vi "Example - Basic IPS-SA Legacy.vi"(0 "Connection Details":T5={"VISA resource name"="", "Comms Layer"=enum."ISOBus - RS-232", "Serial Configuration"={"Baud Rate"=115200, "Parity"=0, "Data Bits"=8, "Stop Bits"=10, "Flow Control"=0}, "ISOBUS address"=-1} {"Serial Configuration"."Flow Control" items=["None", "XON/XOFF", "RTS/CTS", "XON/XOFF & RTS/CTS", "DTR/DSR", "XON/XOFF & DTR/DSR"]; "Serial Configuration"."Stop Bits" items=["1.0"=10, "2.0"=20]; "Serial Configuration"."Data Bits" items=["7"=7, "8"=8]; "Serial Configuration"."Parity" items=["None", "Odd", "Even"]; "Serial Configuration"."Baud Rate" items=["300"=300, "600"=600, "1200"=1200, "2400"=2400, "4800"=4800, "9600"=9600, "14400"=14400, "19200"=19200, "38400"=38400, "57600"=57600, "115200"=115200]}, 4 "stop":bool, 6 "Ramp Controls":T6 {"Target Rate (T/min)" format="%_5g"; "Target Field (T)" format="%_5g"; "Target Rate (A/min)" format="%_5g"; "Target Current (A)" format="%_5g"}, 7 "Display Units":bool caption="AMP/TESLA", 8 "Magnet Controls":T7, 9 "SWITCH\nHEATER":bool, 11 "Sw Delay (s)":dbl=30.0 caption="Time Target (s)") -> (13 "SW HTR\nCONFIRM":bool, 14 "Output Current (A)":dbl format="%.4g", 15 "Magnet Current (A)":dbl format="%.4g", 16 "Output Voltage (V)":dbl format="%.4f", 19 "error out":errorcluster)   [LabVIEW 2013]
uses:
  <instrlib>/Mercury iXX/Public/Controls/Comms Transport Layer.ctl
  <instrlib>/Mercury iXX/Public/Controls/Serial Settings.ctl
  <instrlib>/Mercury iXX/Public/Controls/ISOBus Address.ctl
  <instrlib>/Mercury iXX/Mercury iXX.lvlib
  <instrlib>/Mercury iXX/Public/Libraries/Temperature/Signals/Read/Temperature (Read).vi
  <instrlib>/Mercury iXX/Public/Libraries/Temperature.lvlib
panel:
  out "Switch TS":timestamp
  out "Sentinel":bool
  in  "Tab Control":T1(tab)
  in  "VISA timeout":u32=1000
  in  "Use VISA?":bool
  in  "Interval between messages (ms)":i16=100
  out "Sys_time_stamp":timestamp
  in  "Secondary address":string="1"
  in  "Primary address":string="22"
  in  "Number of units":dbl=1.0 min=1.0 max=10.0 step=1.0 format="%#.0g"
  in  "Level Card?":bool caption="AMP/TESLA"
  out "N2 Level (%)":dbl format="%.1g"
  out "He Level (%)":dbl format="%.1g"
  out "Mode":string
  out "Voltage (V)":dbl(knob) scale=-10.0..10.0
  out "Current (A)":dbl(knob) scale=-60.0..60.0
  out "Elapsed\nTime (s)":dbl caption="Elapsed Time (s)"
  out "Magnet Centre Field (T)":dbl format="%.4f"
  out "Output (T) (Field equivalent)":dbl format="%.4f"
  out "Status":string
  in  "Log file:":string="C:\\temp\\iPS_data.lvm"
  in  "Log Data?":bool
  in  "Plot Data?":bool
  out "Waveform Chart":T8(graph)
  # "Switch Controls"
  # "MercuryiPS-Legacy-VI"
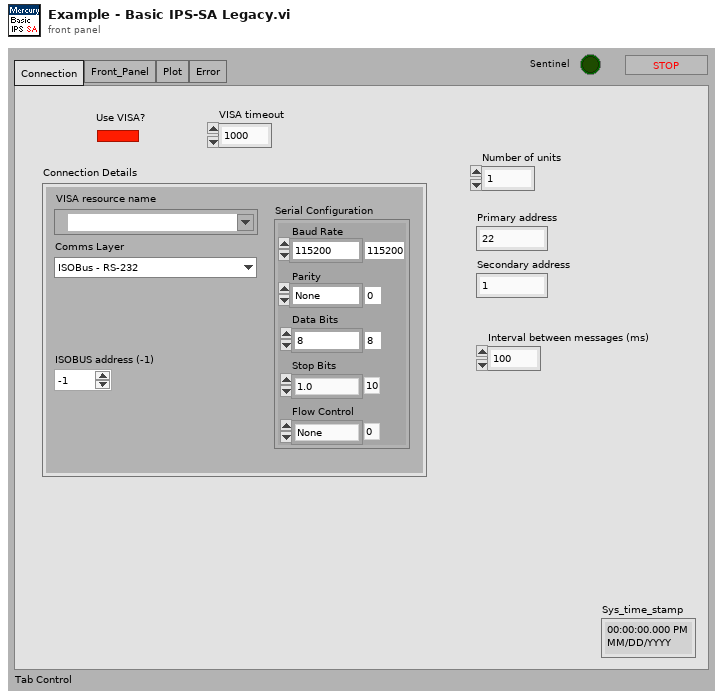
[diagram p1: front panel]
types:
  T1 = enum32{"Connection", "Front_Panel", "Plot", "Error"}
  T2 = typedef "Mercury iXX.lvlib/Comms Transport Layer.ctl" = enum16{"Ethernet TCP/IP", "USB", "ISOBus - RS-232", "GPIB"}
  T3 = typedef "Mercury iXX.lvlib/Serial Settings.ctl" = cluster{"Baud Rate":u32, "Parity":u16, "Data Bits":u16, "Stop Bits":u16, "Flow Control":u16}
  T4 = typedef "Mercury iXX.lvlib/ISOBus Address.ctl" = i32
  T5 = cluster{"VISA resource name":refnum<visa-resource-name>, "Comms Layer":T2, "Serial Configuration":T3, "ISOBUS address":T4}
  T6 = cluster{"Target Current (A)":dbl, "Target Rate (A/min)":dbl, "Target Field (T)":dbl, "Target Rate (T/min)":dbl}
  T7 = cluster{"CLAMP":bool, "HOLD":bool, "TO SET":bool, "TO ZERO":bool}
  T8 = cluster{"Current":dbl, "Persistant Current":dbl, "Voltage":dbl, "Temperature":dbl}
  T9 = cluster{"Current (A) 2":dbl, "Magnet Current (A) 2":dbl, "Voltage (V) 2":dbl, "Temperature":dbl}
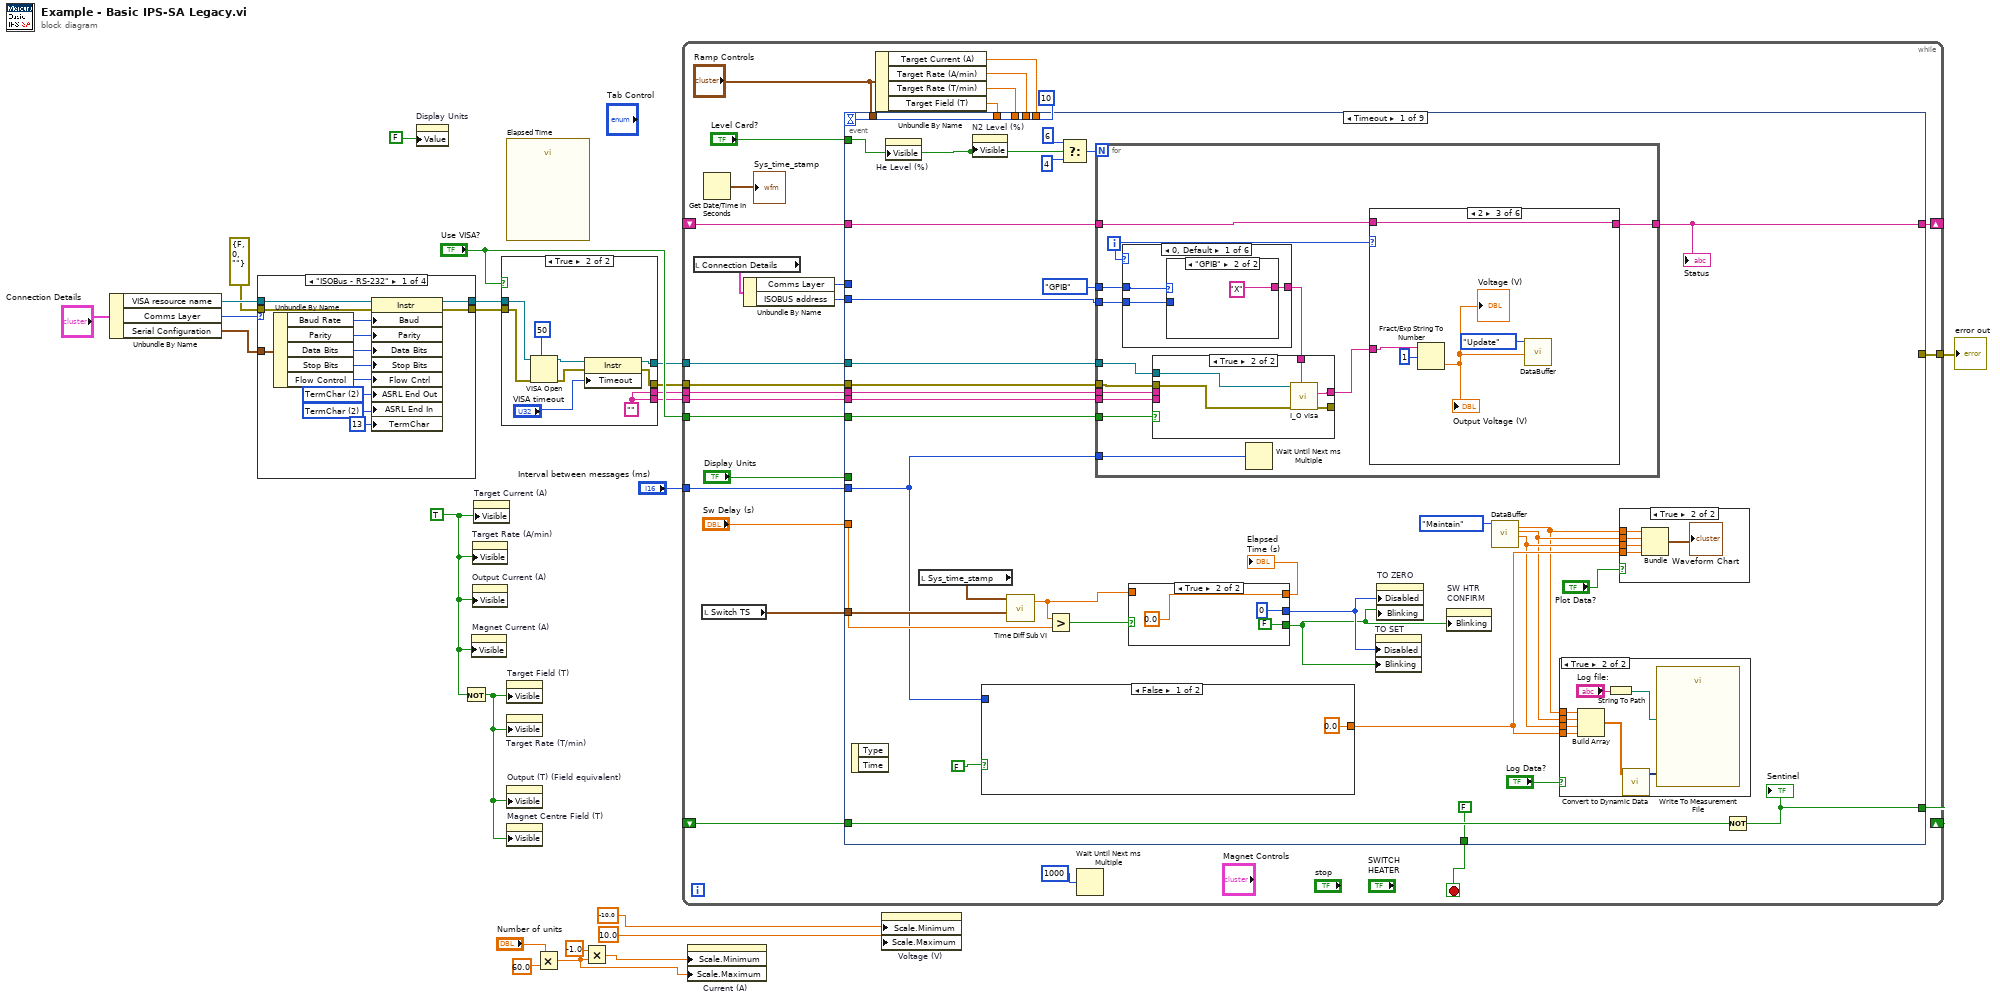
[diagram p0: block diagram]
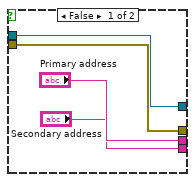
[diagram p2: hidden frame]
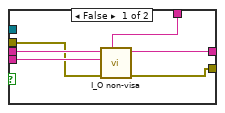
[diagram p6: hidden frame]
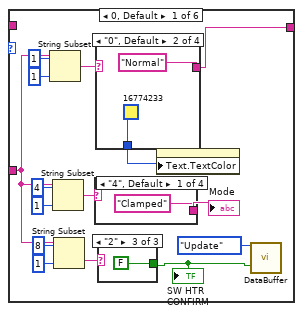
[diagram p7: hidden frame]
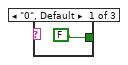
[diagram p8: hidden frame]
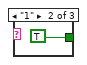
[diagram p9: hidden frame]
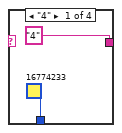
[diagram p10: hidden frame]
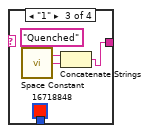
[diagram p11: hidden frame]
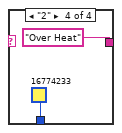
[diagram p12: hidden frame]
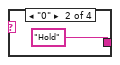
[diagram p13: hidden frame]
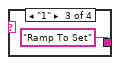
[diagram p14: hidden frame]
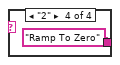
[diagram p15: hidden frame]
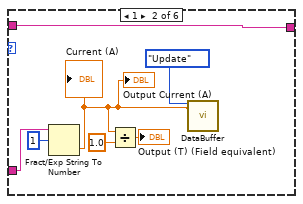
[diagram p16: hidden frame]
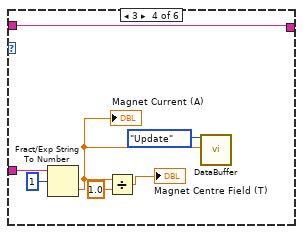
[diagram p17: hidden frame]
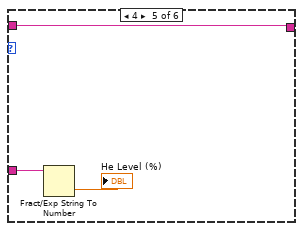
[diagram p18: hidden frame]
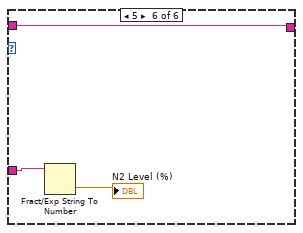
[diagram p19: hidden frame]
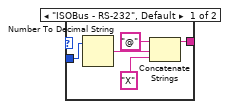
[diagram p20: hidden frame]
diagram:
  w23 = TRUE ("Visible")
  n1 = Unbundle By Name("Connection Details") -> ("VISA resource name"=w13:refnum<visa-resource-name>, "Comms Layer"=w15:T2, "Serial Configuration"=w14:T3)
  n2 = case shown="\"ISOBus - RS-232\"" w15 {
    tunnel: w14 -> [w36 _ _ _]
    tunnel: w13 -> [w37 w39 w41 w43]
    tunnel: errorcluster {"status"=FALSE, "code"=0, "source"=""} ("error in (no error)") -> [w28 w38 w40 w42]
    tunnel: [w27 w39 w41 w43] -> w10
    tunnel: [w26 w38 w40 w42] -> w9
    frame "ISOBus - RS-232" {
      w29 = u16 2 items=["None", "Last Bit", "TermChar"] ("Serial Settings:End Mode for Reads")
      w30 = u16 2 items=["None", "Last Bit", "TermChar", "Break"] ("Serial Settings:End Mode for Writes")
      n3 = Unbundle By Name(w36) -> ("Baud Rate"=w35:u32, "Parity"=w34:u16, "Data Bits"=w33:u16, "Stop Bits"=w32:u16, "Flow Control"=w31:u16)
      n4 = property class="Instr"(reference=w37, error in=w28, "Baud"=w35, "Parity"=w34, "Data Bits"=w33, "Stop Bits"=w32, "Flow Cntrl"=w31, "ASRL End Out"=w30, "ASRL End In"=w29, "TermChar"=u8 13 ("Message Based Settings:Termination Character")) -> (reference out=w27:refnum<visa-resource-name>, error out=w26:errorcluster)
    }
    frame "USB" {
    }
    frame "Ethernet TCP/IP" {
    }
    frame "GPIB" {
    }
  }
  n5 = property on="Display Units" class="Bool (strict)"("Value"=FALSE ("AMP/TESLA")) -> ()  [unwired: 2 in, 2 out]
  n6 = Not(x=w23) -> (.not. x?=w22:bool)
  n7 = property on="Magnet Current (A)" class="DigNum (strict)"("Visible"=w23) -> ()  [unwired: 2 in, 2 out]
  n8 = property on="Target Rate (A/min)" class="DigNum (strict)"("Visible"=w23) -> ()  [unwired: 2 in, 2 out]
  n9 = property on="Output Current (A)" class="DigNum (strict)"("Visible"=w23) -> ()  [unwired: 2 in, 2 out]
  n10 = property on="Target Current (A)" class="DigNum (strict)"("Visible"=w23) -> ()  [unwired: 2 in, 2 out]
  n11 = case shown="True" "Use VISA?" {
    tunnel: w10 -> [w47 w56]
    tunnel: w9 -> [w46 w55]
    tunnel: [w47 w50] -> w5
    tunnel: [w46 w49] -> w6
    tunnel: ["Primary address" w54] -> w8
    tunnel: ["Secondary address" w54] -> w7
    frame False {
    }
    frame True {
      w54 = ""
      n12 = VISA Open(timeout (0)=u32 50 ("VISA Open timeout (0)"), error in (no error)=w55, VISA resource name=w56) -> (VISA resource name=w53:refnum<visa-resource-name>, error out=w52:errorcluster)  [unwired: 2 in]
      n13 = property class="Instr"(reference=w53, error in=w52, "Timeout"="VISA timeout") -> (reference out=w50:refnum<visa-resource-name>, error out=w49:errorcluster)
    }
  }
  n14 = call "Elapsed Time"() -> ()  [unwired: 12 in, 8 out]
  n15 = property on="Target Field (T)" class="DigNum (strict)"("Visible"=w22) -> ()  [unwired: 2 in, 2 out]
  n16 = property on="Target Rate (T/min)" class="DigNum (strict)"("Visible"=w22) -> ()  [unwired: 2 in, 2 out]
  n17 = property on="Output (T) (Field equivalent)" class="DigNum (strict)"("Visible"=w22) -> ()  [unwired: 2 in, 2 out]
  n18 = property on="Magnet Centre Field (T)" class="DigNum (strict)"("Visible"=w22) -> ()  [unwired: 2 in, 2 out]
  n19 = Multiply(x="Number of units", y=60.0) -> (x*y=w18:dbl)
  n20 = Multiply(x=-1.0, y=w18) -> (x*y=w19:dbl)
  n21 = while {
    shift-right: [w80] -> _
    shift-left: _ -> [w81]
    tunnel: [w78] -> w4
    tunnel: "Interval between messages (ms)" -> [w71]
    shift-right: [w66] -> _
    shift-left: _ -> [w70]
    tunnel: "Use VISA?" -> [w65]
    tunnel: w7 -> [w64]
    tunnel: w8 -> [w63]
    tunnel: w6 -> [w62]
    tunnel: w5 -> [w61]
    stop <- w79 stop-if-true
    n22 = local read "Connection Details"() -> (w60:T5)
    n23 = local read "Switch TS"() -> (w69:timestamp)
    n24 = Get Date/Time In Seconds() -> (seconds since 1Jan1904=→"Sys_time_stamp":timestamp)
    n25 = Unbundle By Name(w60) -> ("Comms Layer"=w59:T2, "ISOBUS address"=w58:T4)
    n26 = Unbundle By Name("Ramp Controls") -> ("Target Current (A)"=w74:dbl, "Target Rate (A/min)"=w75:dbl, "Target Rate (T/min)"=w73:dbl, "Target Field (T)"=w72:dbl)
    n27 = event shown="[0] Timeout" {
      selector: _ -> [_ _ _ _ _ _ _ _ _]
      dyn-events: _ -> [_ _ _ _ _ _ _ _ _]
      timeout: 10 -> [_ _ _ _ _ _ _ _ _]
      tunnel: w81 -> [w116 w294 w342 w390 w438 w486 w541 w775 _]
      tunnel: [w115 w294 w342 w390 w438 w486 w541 w775 _] -> w80
      tunnel: [_ _ _ _ _ _ _ _ w780] -> w78
      tunnel: [FALSE FALSE FALSE FALSE FALSE FALSE FALSE TRUE _] -> w79
      tunnel: "Sw Delay (s)" -> [w113 _ _ _ _ _ _ _ _]
      tunnel: "Display Units" -> [_ _ _ _ _ _ w540 _ w779]
      tunnel: w75 -> [_ _ _ _ _ _ w539 _ _]
      tunnel: w74 -> [_ _ _ _ _ _ w538 _ _]
      tunnel: w73 -> [_ _ _ _ _ _ w537 _ _]
      tunnel: w72 -> [_ _ _ _ _ _ w536 _ _]
      tunnel: w71 -> [w96 w291 w333 w381 w429 w484 w535 _ _]
      tunnel: w70 -> [w100 _ _ _ _ _ _ _ _]
      tunnel: w69 -> [w105 _ _ _ _ _ _ _ _]
      tunnel: "Ramp Controls" -> [_ _ _ _ _ _ w534 _ _]
      tunnel: "Level Card?" -> [w93 _ _ _ _ _ _ _ _]
      tunnel: [w101 _ _ _ _ _ _ _ _] -> w66
      tunnel: w65 -> [w99 w285 w334 w382 w430 w474 w530 _ _]
      tunnel: w64 -> [w98 w283 w331 w379 w427 w473 w528 _ _]
      tunnel: w63 -> [w97 w281 w329 w377 w425 w472 w529 _ _]
      tunnel: w62 -> [w95 _ _ _ _ _ _ _ w777]
      tunnel: w61 -> [w94 w279 w327 w375 w423 w471 w527 _ _]
      tunnel: w59 -> [_ w290 w336 w384 w432 w476 w532 _ _]
      tunnel: w58 -> [w85 w287 w335 w383 w431 w475 w531 _ _]
      event Timeout {
        n28 = event-data() -> ()  [unwired: 3 out]
        n29 = property on="He Level (%)" class="DigNum (strict)"("Visible"=w93) -> ()  [unwired: 2 in, 2 out]
        n30 = local read "Sys_time_stamp"() -> (w103:timestamp)
        n31 = property on="N2 Level (%)" class="DigNum (strict)"("Visible"=w93) -> ()  [unwired: 2 in, 2 out]
        n32 = case shown="False" FALSE {
          tunnel: [0.0 ("Temperature") w255] -> w106
          tunnel: w96 -> [_ w253]
          frame False {
          }
          frame True {
            n33 = flat-sequence {
              tunnel: w253 -> [w256]
              tunnel: [w257] -> w254
              tunnel: [w259] -> w255
              tunnel: w254 -> [w259]
              tunnel: w253 -> [w258]
              frame #0 {
                n34 = Wait (ms)(milliseconds to wait=w256) -> ()  [unwired: 1 out]
              }
              frame #1 {
                n35 = call-poly <instrlib>:"Signals (Read).vi"() -> ("Temperature"=w257:dbl)  [unwired: 7 in, 4 out]
              }
              frame #2 {
                n36 = Wait (ms)(milliseconds to wait=w258) -> ()  [unwired: 1 out]
              }
            }
          }
        }
        n37 = call <instrlib>:"Time Diff Sub VI.vi"("Start Time Stamp"=w105, "Current Time Stamp"=w103) -> ("Time Diff"=w104:dbl)  [unwired: 2 in, 1 out]
        n38 = Greater?(x=w104, y=w113) -> (0:w112:bool)
        n39 = Select(t=6, s=w93, f=4) -> (s? t:f=w90:i32)
        n40 = for {
          N: w90 -> [_]
          tunnel: [w126] -> w101
          tunnel: w100 -> [w125]
          tunnel: w99 -> [w124]
          tunnel: w98 -> [w123]
          tunnel: w97 -> [w122]
          tunnel: w96 -> [w121]
          tunnel: w95 -> [w120]
          tunnel: w94 -> [w119]
          tunnel: Comms_Transport_Layer."GPIB" ("Comms Layer") -> [w118]
          tunnel: w85 -> [w117]
          i -> [w128]
          n41 = case shown="0, Default" w128 {
            tunnel: [w199 w207 w218 w225 w234 w244] -> w129
            tunnel: w118 -> [w198 w209 w217 w227 w236 w245]
            tunnel: w117 -> [w200 w208 w216 w226 w235 w243]
            frame 0, Default {
              n42 = case shown="\"GPIB\"" w198 {
                tunnel: [w201 "X" ("data to write")] -> w199
                tunnel: w200 -> [w203 _]
                frame "ISOBus - RS-232", Default {
                  n43 = Number To Decimal String(number=w203) -> (decimal integer string=w204:string)  [unwired: 1 in]
                  n44 = Concatenate Strings("@" ("string"), w204, "X" ("data to write")) -> (w201:string)
                }
                frame "GPIB" {
                }
              }
            }
            frame 1 {
              n45 = case shown="\"ISOBus - RS-232\", Default" w209 {
                tunnel: [w210 "R0" ("data to write")] -> w207
                tunnel: w208 -> [w212 _]
                frame "ISOBus - RS-232", Default {
                  n46 = Number To Decimal String(number=w212) -> (decimal integer string=w213:string)  [unwired: 1 in]
                  n47 = Concatenate Strings("@" ("string"), w213, "R0" ("data to write")) -> (w210:string)
                }
                frame "GPIB" {
                }
              }
            }
            frame 2 {
              n48 = case shown="\"ISOBus - RS-232\", Default" w217 {
                tunnel: [w219 "R1" ("data to write")] -> w218
                tunnel: w216 -> [w221 _]
                frame "ISOBus - RS-232", Default {
                  n49 = Number To Decimal String(number=w221) -> (decimal integer string=w222:string)  [unwired: 1 in]
                  n50 = Concatenate Strings("@" ("string"), w222, "R1" ("data to write")) -> (w219:string)
                }
                frame "GPIB" {
                }
              }
            }
            frame 3 {
              n51 = case shown="\"ISOBus - RS-232\", Default" w227 {
                tunnel: [w228 "R2" ("data to write")] -> w225
                tunnel: w226 -> [w230 _]
                frame "ISOBus - RS-232", Default {
                  n52 = Number To Decimal String(number=w230) -> (decimal integer string=w231:string)  [unwired: 1 in]
                  n53 = Concatenate Strings("@" ("string"), w231, "R2" ("data to write")) -> (w228:string)
                }
                frame "GPIB" {
                }
              }
            }
            frame 4 {
              n54 = case shown="\"GPIB\"" w236 {
                tunnel: [w237 "R10" ("data to write")] -> w234
                tunnel: w235 -> [w239 _]
                frame "ISOBus - RS-232", Default {
                  n55 = Number To Decimal String(number=w239) -> (decimal integer string=w240:string)  [unwired: 1 in]
                  n56 = Concatenate Strings("@" ("string"), w240, "R10" ("data to write")) -> (w237:string)
                }
                frame "GPIB" {
                }
              }
            }
            frame 5 {
              n57 = case shown="\"GPIB\"" w245 {
                tunnel: [w246 "R11" ("data to write")] -> w244
                tunnel: w243 -> [w248 _]
                frame "ISOBus - RS-232", Default {
                  n58 = Number To Decimal String(number=w248) -> (decimal integer string=w249:string)  [unwired: 1 in]
                  n59 = Concatenate Strings("@" ("string"), w249, "R11" ("data to write")) -> (w246:string)
                }
                frame "GPIB" {
                }
              }
            }
          }
          n60 = case shown="True" w124 {
            tunnel: w129 -> [w135 w140]
            tunnel: [w134 w139] -> w127
            tunnel: w123 -> [w133 _]
            tunnel: w122 -> [w132 _]
            tunnel: w120 -> [w130 w138]
            tunnel: w119 -> [_ w137]
            tunnel: [w131 w136] -> _
            frame False {
              n61 = call <instrlib>:"I_O non-visa.vi"("data to write"=w135, "error in"=w130, "Secondary address"=w133, "Primary address"=w132) -> ("error out"=w131:errorcluster, "read data"=w134:string)  [unwired: 6 in]
            }
            frame True {
              n62 = call <instrlib>:"I_O visa.vi"("data to write"=w140, "error in"=w138, "VISA resource name"=w137) -> ("error out"=w136:errorcluster, "read data"=w139:string)  [unwired: 6 in, 1 out]
            }
          }
          n63 = Wait Until Next ms Multiple(millisecond multiple=w121) -> ()  [unwired: 1 out]
          n64 = case shown="2" w128 {
            tunnel: w127 -> [w146 w179 w184 w190 w194 w197]
            tunnel: [w143 w176 w183 w188 w192 w195] -> w126
            tunnel: w125 -> [_ w176 w183 w188 w192 w195]
            frame 0, Default {
              n65 = String Subset(string=w146, offset (0)=1, length (rest)=1 ("length (rest)")) -> (substring=w149:string)
              n66 = String Subset(string=w146, offset (0)=4, length (rest)=1 ("length (rest)")) -> (substring=w151:string)
              n67 = String Subset(string=w146, offset (0)=8, length (rest)=1 ("length (rest)")) -> (substring=w145:string)
              n68 = case shown="\"4\", Default" w151 {
                tunnel: ["Clamped" "Hold" "Ramp To Set" "Ramp To Zero"] -> w150
                frame "4", Default {
                }
                frame "0" {
                }
                frame "1" {
                }
                frame "2" {
                }
              }
              "Mode" <- w150
              n69 = case shown="\"0\", Default" w149 {
                tunnel: ["4" "Normal" w164 "Over Heat"] -> w143
                tunnel: [u32 16774233 ("Text.Text Colors:Text Color") u32 16774233 ("Text.Text Colors:Text Color") u32 16718848 ("Text.Text Colors:Text Color") u32 16774233 ("Text.Text Colors:Text Color")] -> w144
                frame "4" {
                }
                frame "0", Default {
                }
                frame "1" {
                  n70 = call <vilib>:"Space Constant.vi"() -> ("String"=w165:string)
                  n71 = Concatenate Strings("Quenched", w165) -> (w164:string)
                }
                frame "2" {
                }
              }
              n72 = case shown="\"2\"" w145 {
                tunnel: [FALSE TRUE FALSE] -> w142
                frame "0", Default {
                }
                frame "1" {
                }
                frame "2" {
                }
              }
              "SW HTR\nCONFIRM" <- w142
              n73 = property on="Status" class="Str"("Text.TextColor"=w144) -> ()  [unwired: 2 in, 2 out]
              n74 = call <instrlib>:"DataBuffer.vi"("Enum"=enum16{"Maintain", "Update", "Initialise"}."Update", "Switch Htr State"=w142) -> ()  [unwired: 14 in, 4 out]
            }
            frame 1 {
              n75 = Fract/Exp String To Number(string=w179, offset=1) -> (number=w173:dbl)  [unwired: 2 in, 1 out]
              "Output Current (A)" <- w173
              "Current (A)" <- w173
              n76 = Divide(x=w173, y=1.0) -> (x/y=→"Output (T) (Field equivalent)":dbl)
              n77 = call <instrlib>:"DataBuffer.vi"("Enum"=enum16{"Maintain", "Update", "Initialise"}."Update", "Current (A)"=w173) -> ()  [unwired: 14 in, 4 out]
            }
            frame 2 {
              n78 = Fract/Exp String To Number(string=w184, offset=1) -> (number=w182:dbl)  [unwired: 2 in, 1 out]
              "Voltage (V)" <- w182
              "Output Voltage (V)" <- w182
              n79 = call <instrlib>:"DataBuffer.vi"("Enum"=enum16{"Maintain", "Update", "Initialise"}."Update", "Voltage (V)"=w182) -> ()  [unwired: 14 in, 4 out]
            }
            frame 3 {
              n80 = Fract/Exp String To Number(string=w190, offset=1) -> (number=w187:dbl)  [unwired: 2 in, 1 out]
              "Magnet Current (A)" <- w187
              n81 = Divide(x=w187, y=1.0) -> (x/y=→"Magnet Centre Field (T)":dbl)
              n82 = call <instrlib>:"DataBuffer.vi"("Enum"=enum16{"Maintain", "Update", "Initialise"}."Update", "Magnet Current (A)"=w187) -> ()  [unwired: 14 in, 4 out]
            }
            frame 4 {
              n83 = Fract/Exp String To Number(string=w194) -> (number=→"He Level (%)":dbl)  [unwired: 3 in, 1 out]
            }
            frame 5 {
              n84 = Fract/Exp String To Number(string=w197) -> (number=→"N2 Level (%)":dbl)  [unwired: 3 in, 1 out]
            }
          }
        }
        "Status" <- w101
        n85 = case shown="True" w112 {
          tunnel: [w275 0.0 ("Elapsed\nTime (s)")] -> w111
          tunnel: w104 -> [w275 _]
          tunnel: [TRUE ("Blinking") FALSE ("Blinking")] -> w109
          tunnel: [u8 1 ("Disabled") u8 0 ("Disabled")] -> w110
          frame False {
          }
          frame True {
          }
        }
        "Elapsed\nTime (s)" <- w111
        n86 = property on="TO SET" class="Bool"("Disabled"=w110, "Blinking"=w109) -> ()  [unwired: 2 in, 2 out]
        n87 = property on="TO ZERO" class="Bool"("Disabled"=w110, "Blinking"=w109) -> ()  [unwired: 2 in, 2 out]
        n88 = property on="SW HTR\nCONFIRM" class="Bool (strict)"("Blinking"=w109) -> ()  [unwired: 2 in, 2 out]
        n89 = call <instrlib>:"DataBuffer.vi"("Enum"=enum16{"Maintain", "Update", "Initialise"}."Maintain") -> ("Current (A) 2"=w86:dbl, "Magnet Current (A) 2"=w87:dbl, "Voltage (V) 2"=w88:dbl)  [unwired: 15 in, 1 out]
        n90 = case shown="True" "Log Data?" {
          tunnel: w106 -> [_ w263]
          tunnel: w88 -> [_ w262]
          tunnel: w87 -> [_ w261]
          tunnel: w86 -> [_ w260]
          frame False {
          }
          frame True {
            n91 = Build Array(w260, w261, w262, w263) -> (w265:dbl[])
            n92 = String To Path(string="Log file:") -> (path=w266:path)
            n93 = call "Convert to Dynamic Data"("Array"=w265) -> ("Dynamic Data Type"=w264:dynamicdata)  [unwired: 3 in]
            n94 = call "Write To Measurement File"("Signals"=w264, "Filename"=w266) -> ()  [unwired: 15 in, 3 out]
          }
        }
        n95 = case shown="True" "Plot Data?" {
          tunnel: w106 -> [_ w272]
          tunnel: w88 -> [_ w271]
          tunnel: w87 -> [_ w270]
          tunnel: w86 -> [_ w269]
          frame False {
          }
          frame True {
            n96 = Bundle("Current (A) 2"=w269, "Magnet Current (A) 2"=w270, "Voltage (V) 2"=w271, "Temperature"=w272) -> (→"Waveform Chart":T9)  [unwired: 1 in]
          }
        }
        n97 = Not(x=w116) -> (.not. x?=w115:bool)
        "Sentinel" <- w115
      }
      event "Magnet Controls.HOLD": Mouse Down {
        n98 = event-data() -> ()  [unwired: 7 out]
        n99 = flat-sequence {
          tunnel: [w302] -> w292
          tunnel: w291 -> [w302]
          tunnel: w290 -> [w301]
          tunnel: [w301] -> w289
          tunnel: [w300] -> w288
          tunnel: w287 -> [w300]
          tunnel: [w299] -> w286
          tunnel: w285 -> [w299]
          tunnel: [w298] -> w284
          tunnel: w283 -> [w298]
          tunnel: [w297] -> w282
          tunnel: w281 -> [w297]
          tunnel: [w296] -> w280
          tunnel: w279 -> [w296]
          tunnel: [w310] -> w293
          tunnel: w292 -> [w310]
          tunnel: w289 -> [w308]
          tunnel: w288 -> [w307]
          tunnel: w286 -> [w306]
          tunnel: w284 -> [w305]
          tunnel: w282 -> [w304]
          tunnel: w280 -> [w303]
          tunnel: w293 -> [w326]
          frame #0 {
            n100 = Wait (ms)(milliseconds to wait=w302) -> ()  [unwired: 1 out]
          }
          frame #1 {
            n101 = case shown="\"ISOBus - RS-232\", Default" w308 {
              tunnel: [w312 "A0" ("data to write")] -> w309
              tunnel: w307 -> [w311 _]
              frame "ISOBus - RS-232", Default {
                n102 = Number To Decimal String(number=w311) -> (decimal integer string=w314:string)  [unwired: 1 in]
                n103 = Concatenate Strings("@" ("string"), w314, "A0" ("data to write")) -> (w312:string)
              }
              frame "GPIB" {
              }
            }
            n104 = case shown="True" w306 {
              tunnel: w309 -> [w321 w325]
              tunnel: [w320 w324] -> _
              tunnel: [w319 w323] -> _
              tunnel: w305 -> [w318 _]
              tunnel: w304 -> [w317 _]
              tunnel: w303 -> [_ w322]
              frame False {
                n105 = call <instrlib>:"I_O non-visa.vi"("data to write"=w321, "Secondary address"=w318, "Primary address"=w317) -> ("error out"=w319:errorcluster, "read data"=w320:string)  [unwired: 7 in]
              }
              frame True {
                n106 = call <instrlib>:"I_O visa.vi"("data to write"=w325, "VISA resource name"=w322) -> ("error out"=w323:errorcluster, "read data"=w324:string)  [unwired: 7 in, 1 out]
              }
            }
          }
          frame #2 {
            n107 = Wait (ms)(milliseconds to wait=w326) -> ()  [unwired: 1 out]
          }
        }
      }
      event "Magnet Controls.CLAMP": Mouse Down {
        n108 = event-data() -> ()  [unwired: 7 out]
        n109 = flat-sequence {
          tunnel: [w350] -> w341
          tunnel: w333 -> [w350]
          tunnel: w336 -> [w349]
          tunnel: [w349] -> w340
          tunnel: [w348] -> w339
          tunnel: w335 -> [w348]
          tunnel: [w347] -> w338
          tunnel: w334 -> [w347]
          tunnel: [w346] -> w332
          tunnel: w331 -> [w346]
          tunnel: [w345] -> w330
          tunnel: w329 -> [w345]
          tunnel: [w344] -> w328
          tunnel: w327 -> [w344]
          tunnel: [w358] -> w337
          tunnel: w341 -> [w358]
          tunnel: w340 -> [w356]
          tunnel: w339 -> [w355]
          tunnel: w338 -> [w354]
          tunnel: w332 -> [w353]
          tunnel: w330 -> [w352]
          tunnel: w328 -> [w351]
          tunnel: w337 -> [w374]
          frame #0 {
            n110 = Wait (ms)(milliseconds to wait=w350) -> ()  [unwired: 1 out]
          }
          frame #1 {
            n111 = case shown="\"GPIB\"" w356 {
              tunnel: [w360 "A4" ("data to write")] -> w357
              tunnel: w355 -> [w359 _]
              frame "ISOBus - RS-232", Default {
                n112 = Number To Decimal String(number=w359) -> (decimal integer string=w362:string)  [unwired: 1 in]
                n113 = Concatenate Strings("@" ("string"), w362, "A4" ("data to write")) -> (w360:string)
              }
              frame "GPIB" {
              }
            }
            n114 = case shown="True" w354 {
              tunnel: w357 -> [w369 w373]
              tunnel: [w368 w372] -> _
              tunnel: [w367 w371] -> _
              tunnel: w353 -> [w366 _]
              tunnel: w352 -> [w365 _]
              tunnel: w351 -> [_ w370]
              frame False {
                n115 = call <instrlib>:"I_O non-visa.vi"("data to write"=w369, "Secondary address"=w366, "Primary address"=w365) -> ("error out"=w367:errorcluster, "read data"=w368:string)  [unwired: 7 in]
              }
              frame True {
                n116 = call <instrlib>:"I_O visa.vi"("data to write"=w373, "VISA resource name"=w370) -> ("error out"=w371:errorcluster, "read data"=w372:string)  [unwired: 7 in, 1 out]
              }
            }
          }
          frame #2 {
            n117 = Wait (ms)(milliseconds to wait=w374) -> ()  [unwired: 1 out]
          }
        }
      }
      event "Magnet Controls.TO SET": Mouse Down {
        n118 = event-data() -> ()  [unwired: 7 out]
        n119 = flat-sequence {
          tunnel: [w398] -> w389
          tunnel: w381 -> [w398]
          tunnel: w384 -> [w397]
          tunnel: [w397] -> w388
          tunnel: [w396] -> w387
          tunnel: w383 -> [w396]
          tunnel: [w395] -> w386
          tunnel: w382 -> [w395]
          tunnel: [w394] -> w380
          tunnel: w379 -> [w394]
          tunnel: [w393] -> w378
          tunnel: w377 -> [w393]
          tunnel: [w392] -> w376
          tunnel: w375 -> [w392]
          tunnel: [w406] -> w385
          tunnel: w389 -> [w406]
          tunnel: w388 -> [w404]
          tunnel: w387 -> [w403]
          tunnel: w386 -> [w402]
          tunnel: w380 -> [w401]
          tunnel: w378 -> [w400]
          tunnel: w376 -> [w399]
          tunnel: w385 -> [w422]
          frame #0 {
            n120 = Wait (ms)(milliseconds to wait=w398) -> ()  [unwired: 1 out]
          }
          frame #1 {
            n121 = case shown="\"ISOBus - RS-232\", Default" w404 {
              tunnel: [w408 "A1" ("data to write")] -> w405
              tunnel: w403 -> [w407 _]
              frame "ISOBus - RS-232", Default {
                n122 = Number To Decimal String(number=w407) -> (decimal integer string=w410:string)  [unwired: 1 in]
                n123 = Concatenate Strings("@" ("string"), w410, "A1" ("data to write")) -> (w408:string)
              }
              frame "GPIB" {
              }
            }
            n124 = case shown="True" w402 {
              tunnel: w405 -> [w417 w421]
              tunnel: [w416 w420] -> _
              tunnel: [w415 w419] -> _
              tunnel: w401 -> [w414 _]
              tunnel: w400 -> [w413 _]
              tunnel: w399 -> [_ w418]
              frame False {
                n125 = call <instrlib>:"I_O non-visa.vi"("data to write"=w417, "Secondary address"=w414, "Primary address"=w413) -> ("error out"=w415:errorcluster, "read data"=w416:string)  [unwired: 7 in]
              }
              frame True {
                n126 = call <instrlib>:"I_O visa.vi"("data to write"=w421, "VISA resource name"=w418) -> ("error out"=w419:errorcluster, "read data"=w420:string)  [unwired: 7 in, 1 out]
              }
            }
          }
          frame #2 {
            n127 = Wait (ms)(milliseconds to wait=w422) -> ()  [unwired: 1 out]
          }
        }
      }
      event "Magnet Controls.TO ZERO": Mouse Down {
        n128 = event-data() -> ()  [unwired: 7 out]
        n129 = flat-sequence {
          tunnel: [w446] -> w437
          tunnel: w429 -> [w446]
          tunnel: w432 -> [w445]
          tunnel: [w445] -> w436
          tunnel: [w444] -> w435
          tunnel: w431 -> [w444]
          tunnel: [w443] -> w434
          tunnel: w430 -> [w443]
          tunnel: [w442] -> w428
          tunnel: w427 -> [w442]
          tunnel: [w441] -> w426
          tunnel: w425 -> [w441]
          tunnel: [w440] -> w424
          tunnel: w423 -> [w440]
          tunnel: [w454] -> w433
          tunnel: w437 -> [w454]
          tunnel: w436 -> [w452]
          tunnel: w435 -> [w451]
          tunnel: w434 -> [w450]
          tunnel: w428 -> [w449]
          tunnel: w426 -> [w448]
          tunnel: w424 -> [w447]
          tunnel: w433 -> [w470]
          frame #0 {
            n130 = Wait (ms)(milliseconds to wait=w446) -> ()  [unwired: 1 out]
          }
          frame #1 {
            n131 = case shown="\"ISOBus - RS-232\", Default" w452 {
              tunnel: [w456 "A2" ("data to write")] -> w453
              tunnel: w451 -> [w455 _]
              frame "ISOBus - RS-232", Default {
                n132 = Number To Decimal String(number=w455) -> (decimal integer string=w458:string)  [unwired: 1 in]
                n133 = Concatenate Strings("@" ("string"), w458, "A2" ("data to write")) -> (w456:string)
              }
              frame "GPIB" {
              }
            }
            n134 = case shown="True" w450 {
              tunnel: w453 -> [w465 w469]
              tunnel: [w464 w468] -> _
              tunnel: [w463 w467] -> _
              tunnel: w449 -> [w462 _]
              tunnel: w448 -> [w461 _]
              tunnel: w447 -> [_ w466]
              frame False {
                n135 = call <instrlib>:"I_O non-visa.vi"("data to write"=w465, "Secondary address"=w462, "Primary address"=w461) -> ("error out"=w463:errorcluster, "read data"=w464:string)  [unwired: 7 in]
              }
              frame True {
                n136 = call <instrlib>:"I_O visa.vi"("data to write"=w469, "VISA resource name"=w466) -> ("error out"=w467:errorcluster, "read data"=w468:string)  [unwired: 7 in, 1 out]
              }
            }
          }
          frame #2 {
            n137 = Wait (ms)(milliseconds to wait=w470) -> ()  [unwired: 1 out]
          }
        }
      }
      event "SWITCH\nHEATER": Mouse Down {
        n138 = event-data() -> ()  [unwired: 2 out]
        n139 = call <instrlib>:"DataBuffer.vi"("Enum"=enum16{"Maintain", "Update", "Initialise"}."Maintain") -> ("Current (A) 2"=w479:dbl, "Magnet Current (A) 2"=w478:dbl)  [unwired: 15 in, 2 out]
        n140 = Subtract(x=w479, y=w478) -> (x-y=w481:dbl)
        n141 = Absolute Value(x=w481) -> (abs(x)=w482:dbl)
        n142 = Less?(x=w482, y=0.1) -> (x < y?=w480:bool)
        n143 = case shown="False" w480 {
          selector: w480 -> [_ w490]
          tunnel: [w489 w490] -> w485
          frame False {
            n144 = Two Button Dialog(message="The magnet current is more\nthan 0.1A different to the\nPSU output current.  It is not\nadvisable to switch on the\nswitch heater unless these\ncurrents are equal!") -> (T button?=w489:bool)  [unwired: 2 out]
          }
          frame True {
          }
        }
        n145 = case shown="True" w485 {
          tunnel: w484 -> [_ w497]
          tunnel: w476 -> [_ w496]
          tunnel: w475 -> [_ w495]
          tunnel: w474 -> [_ w494]
          tunnel: w473 -> [_ w493]
          tunnel: w472 -> [_ w492]
          tunnel: w471 -> [_ w491]
          frame False {
          }
          frame True {
            n146 = flat-sequence {
              tunnel: w496 -> [w503]
              tunnel: w495 -> [w502]
              tunnel: w494 -> [w501]
              tunnel: w493 -> [w500]
              tunnel: w492 -> [w499]
              tunnel: w491 -> [w498]
              tunnel: w497 -> [w525]
              frame #0 {
                n147 = call <instrlib>:"DataBuffer.vi"("Enum"=enum16{"Maintain", "Update", "Initialise"}."Maintain") -> ("Sw Htr State 2"=w508:bool)  [unwired: 15 in, 3 out]
                n148 = Select(t="H0" ("data to write"), s=w508, f="H2" ("data to write")) -> (s? t:f=w505:string)
                n149 = case shown="\"ISOBus - RS-232\", Default" w503 {
                  tunnel: [w512 w515] -> w504
                  tunnel: w505 -> [w511 w515]
                  tunnel: w502 -> [w510 _]
                  frame "ISOBus - RS-232", Default {
                    n150 = Number To Decimal String(number=w510) -> (decimal integer string=w514:string)  [unwired: 1 in]
                    n151 = Concatenate Strings("@" ("string"), w514, w511) -> (w512:string)
                  }
                  frame "GPIB" {
                  }
                }
                n152 = case shown="True" w501 {
                  tunnel: [w520 w524] -> _
                  tunnel: [w519 w523] -> _
                  tunnel: w504 -> [w518 w522]
                  tunnel: w500 -> [w516 _]
                  tunnel: w499 -> [w517 _]
                  tunnel: w498 -> [_ w521]
                  frame False {
                    n153 = call <instrlib>:"I_O non-visa.vi"("data to write"=w518, "Secondary address"=w516, "Primary address"=w517) -> ("error out"=w519:errorcluster, "read data"=w520:string)  [unwired: 7 in]
                  }
                  frame True {
                    n154 = call <instrlib>:"I_O visa.vi"("data to write"=w522, "VISA resource name"=w521) -> ("error out"=w523:errorcluster, "read data"=w524:string)  [unwired: 7 in, 1 out]
                  }
                }
              }
              frame #1 {
                n155 = Wait (ms)(milliseconds to wait=w525) -> ()  [unwired: 1 out]
              }
              frame #2 {
                n156 = local read "Sys_time_stamp"() -> (→"Switch TS":timestamp)
              }
            }
          }
        }
      }
      event "Ramp Controls": Value Change {
        n157 = event-data() -> ()  [unwired: 6 out]
        n158 = case shown="False" w540 {
          tunnel: w539 -> [w572 _]
          tunnel: w538 -> [w573 _]
          tunnel: w537 -> [_ w673]
          tunnel: w536 -> [_ w674]
          tunnel: w535 -> [w575 w675]
          tunnel: w534 -> [w570 w694]
          tunnel: [w569 w693] -> w533
          tunnel: w532 -> [w567 w677]
          tunnel: w531 -> [w565 w678]
          tunnel: w530 -> [w563 w676]
          tunnel: w529 -> [w553 w671]
          tunnel: w528 -> [w551 w669]
          tunnel: w527 -> [w555 w667]
          frame False {
            n159 = Divide(x=w573, y=1.0) -> (x/y=w574:dbl)
            n160 = Divide(x=w572, y=1.0) -> (x/y=w571:dbl)
            n161 = flat-sequence {
              tunnel: w573 -> [w588]
              tunnel: [w588] -> w580
              tunnel: [w587] -> w576
              tunnel: w575 -> [w587]
              tunnel: [w586] -> w568
              tunnel: w567 -> [w586]
              tunnel: [w585] -> w566
              tunnel: w565 -> [w585]
              tunnel: [w584] -> w564
              tunnel: w563 -> [w584]
              tunnel: [w583] -> w556
              tunnel: w555 -> [w583]
              tunnel: [w582] -> w554
              tunnel: w553 -> [w582]
              tunnel: [w581] -> w552
              tunnel: w551 -> [w581]
              tunnel: w580 -> [w595]
              tunnel: [w597] -> w577
              tunnel: w576 -> [w597]
              tunnel: w568 -> [w593]
              tunnel: w566 -> [w592]
              tunnel: w564 -> [w594]
              tunnel: [w594] -> w561
              tunnel: [w593] -> w559
              tunnel: [w592] -> w557
              tunnel: w556 -> [w589]
              tunnel: w554 -> [w590]
              tunnel: w552 -> [w591]
              tunnel: [w591] -> w549
              tunnel: [w590] -> w547
              tunnel: [w589] -> w545
              tunnel: [w626] -> w578
              tunnel: w577 -> [w626]
              tunnel: [w625] -> w562
              tunnel: w561 -> [w625]
              tunnel: [w624] -> w560
              tunnel: w559 -> [w624]
              tunnel: [w623] -> w558
              tunnel: w557 -> [w623]
              tunnel: [w622] -> w550
              tunnel: w549 -> [w622]
              tunnel: [w621] -> w548
              tunnel: w547 -> [w621]
              tunnel: [w620] -> w546
              tunnel: w545 -> [w620]
              tunnel: w572 -> [w634]
              tunnel: [w635] -> w579
              tunnel: w578 -> [w635]
              tunnel: w562 -> [w633]
              tunnel: w560 -> [w632]
              tunnel: w558 -> [w631]
              tunnel: w550 -> [w629]
              tunnel: w548 -> [w628]
              tunnel: w546 -> [w627]
              tunnel: w579 -> [w658]
              frame #0 {
                n162 = Wait (ms)(milliseconds to wait=w587) -> ()  [unwired: 1 out]
              }
              frame #1 {
                n163 = case shown="\"ISOBus - RS-232\", Default" w593 {
                  tunnel: [w603 w606] -> w596
                  tunnel: w592 -> [w602 _]
                  tunnel: w595 -> [w600 w609]
                  frame "ISOBus - RS-232", Default {
                    n164 = Number To Decimal String(number=w602) -> (decimal integer string=w605:string)  [unwired: 1 in]
                    n165 = Number To Fractional String(number=w600, precision (6)=i16 4) -> (F-format string=w598:string)  [unwired: 2 in]
                    n166 = Concatenate Strings("@" ("string"), w605, "I" ("data to write"), w598) -> (w603:string)
                  }
                  frame "GPIB" {
                    n167 = Number To Fractional String(number=w609, precision (6)=i16 4) -> (F-format string=w607:string)  [unwired: 2 in]
                    n168 = Concatenate Strings("I" ("data to write"), w607) -> (w606:string)
                  }
                }
                n169 = case shown="True" w594 {
                  tunnel: w596 -> [w615 w619]
                  tunnel: [w614 w618] -> _
                  tunnel: [w613 w617] -> _
                  tunnel: w591 -> [w612 _]
                  tunnel: w590 -> [w611 _]
                  tunnel: w589 -> [_ w616]
                  frame False {
                    n170 = call <instrlib>:"I_O non-visa.vi"("data to write"=w615, "Secondary address"=w612, "Primary address"=w611) -> ("error out"=w613:errorcluster, "read data"=w614:string)  [unwired: 7 in]
                  }
                  frame True {
                    n171 = call <instrlib>:"I_O visa.vi"("data to write"=w619, "VISA resource name"=w616) -> ("error out"=w617:errorcluster, "read data"=w618:string)  [unwired: 7 in, 1 out]
                  }
                }
              }
              frame #2 {
                n172 = Wait (ms)(milliseconds to wait=w626) -> ()  [unwired: 1 out]
              }
              frame #3 {
                n173 = case shown="\"GPIB\"" w632 {
                  tunnel: [w641 w644] -> w630
                  tunnel: w631 -> [w640 _]
                  tunnel: w634 -> [w638 w647]
                  frame "ISOBus - RS-232", Default {
                    n174 = Number To Decimal String(number=w640) -> (decimal integer string=w643:string)  [unwired: 1 in]
                    n175 = Number To Fractional String(number=w638, precision (6)=i16 4) -> (F-format string=w636:string)  [unwired: 2 in]
                    n176 = Concatenate Strings("@" ("string"), w643, "S" ("data to write"), w636) -> (w641:string)
                  }
                  frame "GPIB" {
                    n177 = Number To Fractional String(number=w647, precision (6)=i16 4) -> (F-format string=w645:string)  [unwired: 2 in]
                    n178 = Concatenate Strings("S" ("data to write"), w645) -> (w644:string)
                  }
                }
                n179 = case shown="True" w633 {
                  tunnel: w630 -> [w653 w657]
                  tunnel: [w652 w656] -> _
                  tunnel: [w651 w655] -> _
                  tunnel: w629 -> [w650 _]
                  tunnel: w628 -> [w649 _]
                  tunnel: w627 -> [_ w654]
                  frame False {
                    n180 = call <instrlib>:"I_O non-visa.vi"("data to write"=w653, "Secondary address"=w650, "Primary address"=w649) -> ("error out"=w651:errorcluster, "read data"=w652:string)  [unwired: 7 in]
                  }
                  frame True {
                    n181 = call <instrlib>:"I_O visa.vi"("data to write"=w657, "VISA resource name"=w654) -> ("error out"=w655:errorcluster, "read data"=w656:string)  [unwired: 7 in, 1 out]
                  }
                }
              }
              frame #4 {
                n182 = Wait (ms)(milliseconds to wait=w658) -> ()  [unwired: 1 out]
              }
            }
            n183 = Bundle By Name(cluster=w570, "Target Field (T)"=w574, "Target Rate (T/min)"=w571) -> (w569:T6)
          }
          frame True {
            n184 = Multiply(x=w674, y=1.0) -> (x*y=w696:dbl)
            n185 = Multiply(x=w673, y=1.0) -> (x*y=w695:dbl)
            n186 = Bundle By Name(cluster=w694, "Target Current (A)"=w696, "Target Rate (A/min)"=w695) -> (w693:T6)
            n187 = flat-sequence {
              tunnel: w674 -> [w704]
              tunnel: [w704] -> w692
              tunnel: [w703] -> w691
              tunnel: w675 -> [w703]
              tunnel: [w702] -> w690
              tunnel: w677 -> [w702]
              tunnel: [w701] -> w689
              tunnel: w678 -> [w701]
              tunnel: [w700] -> w688
              tunnel: w676 -> [w700]
              tunnel: w671 -> [w699]
              tunnel: [w699] -> w672
              tunnel: [w698] -> w670
              tunnel: w669 -> [w698]
              tunnel: [w697] -> w668
              tunnel: w667 -> [w697]
              tunnel: w692 -> [w711]
              tunnel: [w713] -> w687
              tunnel: w691 -> [w713]
              tunnel: w690 -> [w709]
              tunnel: w689 -> [w708]
              tunnel: w688 -> [w710]
              tunnel: [w710] -> w686
              tunnel: [w709] -> w685
              tunnel: [w708] -> w684
              tunnel: w672 -> [w706]
              tunnel: w670 -> [w707]
              tunnel: w668 -> [w705]
              tunnel: [w707] -> w665
              tunnel: [w706] -> w663
              tunnel: [w705] -> w661
              tunnel: [w742] -> w683
              tunnel: w687 -> [w742]
              tunnel: [w741] -> w682
              tunnel: w686 -> [w741]
              tunnel: [w740] -> w681
              tunnel: w685 -> [w740]
              tunnel: [w739] -> w680
              tunnel: w684 -> [w739]
              tunnel: [w738] -> w666
              tunnel: w665 -> [w738]
              tunnel: [w737] -> w664
              tunnel: w663 -> [w737]
              tunnel: [w736] -> w662
              tunnel: w661 -> [w736]
              tunnel: w673 -> [w750]
              tunnel: [w751] -> w679
              tunnel: w683 -> [w751]
              tunnel: w682 -> [w749]
              tunnel: w681 -> [w748]
              tunnel: w680 -> [w747]
              tunnel: w666 -> [w744]
              tunnel: w664 -> [w745]
              tunnel: w662 -> [w743]
              tunnel: w679 -> [w774]
              frame #0 {
                n188 = Wait (ms)(milliseconds to wait=w703) -> ()  [unwired: 1 out]
              }
              frame #1 {
                n189 = case shown="\"GPIB\"" w709 {
                  tunnel: [w719 w722] -> w712
                  tunnel: w708 -> [w718 _]
                  tunnel: w711 -> [w716 w725]
                  frame "ISOBus - RS-232", Default {
                    n190 = Number To Decimal String(number=w718) -> (decimal integer string=w721:string)  [unwired: 1 in]
                    n191 = Number To Fractional String(number=w716, precision (6)=i16 4) -> (F-format string=w714:string)  [unwired: 2 in]
                    n192 = Concatenate Strings("@" ("string"), w721, "J" ("data to write"), w714) -> (w719:string)
                  }
                  frame "GPIB" {
                    n193 = Number To Fractional String(number=w725, precision (6)=i16 4) -> (F-format string=w723:string)  [unwired: 2 in]
                    n194 = Concatenate Strings("J" ("data to write"), w723) -> (w722:string)
                  }
                }
                n195 = case shown="True" w710 {
                  tunnel: w712 -> [w731 w735]
                  tunnel: [w730 w734] -> _
                  tunnel: [w729 w733] -> _
                  tunnel: w706 -> [w728 _]
                  tunnel: w707 -> [w727 _]
                  tunnel: w705 -> [_ w732]
                  frame False {
                    n196 = call <instrlib>:"I_O non-visa.vi"("data to write"=w731, "Secondary address"=w727, "Primary address"=w728) -> ("error out"=w729:errorcluster, "read data"=w730:string)  [unwired: 7 in]
                  }
                  frame True {
                    n197 = call <instrlib>:"I_O visa.vi"("data to write"=w735, "VISA resource name"=w732) -> ("error out"=w733:errorcluster, "read data"=w734:string)  [unwired: 7 in, 1 out]
                  }
                }
              }
              frame #2 {
                n198 = Wait (ms)(milliseconds to wait=w742) -> ()  [unwired: 1 out]
              }
              frame #3 {
                n199 = case shown="\"ISOBus - RS-232\", Default" w748 {
                  tunnel: [w757 w760] -> w746
                  tunnel: w747 -> [w756 _]
                  tunnel: w750 -> [w754 w763]
                  frame "ISOBus - RS-232", Default {
                    n200 = Number To Decimal String(number=w756) -> (decimal integer string=w759:string)  [unwired: 1 in]
                    n201 = Number To Fractional String(number=w754, precision (6)=i16 4) -> (F-format string=w752:string)  [unwired: 2 in]
                    n202 = Concatenate Strings("@" ("string"), w759, "T" ("data to write"), w752) -> (w757:string)
                  }
                  frame "GPIB" {
                    n203 = Number To Fractional String(number=w763, precision (6)=i16 4) -> (F-format string=w761:string)  [unwired: 2 in]
                    n204 = Concatenate Strings("T" ("data to write"), w761) -> (w760:string)
                  }
                }
                n205 = case shown="True" w749 {
                  tunnel: w746 -> [w769 w773]
                  tunnel: [w768 w772] -> _
                  tunnel: [w767 w771] -> _
                  tunnel: w745 -> [w765 _]
                  tunnel: w744 -> [w766 _]
                  tunnel: w743 -> [_ w770]
                  frame False {
                    n206 = call <instrlib>:"I_O non-visa.vi"("data to write"=w769, "Secondary address"=w766, "Primary address"=w765) -> ("error out"=w767:errorcluster, "read data"=w768:string)  [unwired: 7 in]
                  }
                  frame True {
                    n207 = call <instrlib>:"I_O visa.vi"("data to write"=w773, "VISA resource name"=w770) -> ("error out"=w771:errorcluster, "read data"=w772:string)  [unwired: 7 in, 1 out]
                  }
                }
              }
              frame #4 {
                n208 = Wait (ms)(milliseconds to wait=w774) -> ()  [unwired: 1 out]
              }
            }
          }
        }
        n209 = local write "Ramp Controls"(w533) -> ()
      }
      event "stop": Mouse Down {
        n210 = event-data() -> ()  [unwired: 2 out]
      }
      event "Display Units": Value Change {
        n211 = event-data() -> ()  [unwired: 6 out]
        n212 = property on="Output (T) (Field equivalent)" class="DigNum (strict)"(error in=w777, "Visible"=w779) -> (error out=w787:errorcluster)  [unwired: 1 in, 1 out]
        n213 = property on="Magnet Centre Field (T)" class="DigNum (strict)"(error in=w787, "Visible"=w779) -> (error out=w786:errorcluster)  [unwired: 1 in, 1 out]
        n214 = property on="Target Rate (T/min)" class="DigNum (strict)"(error in=w786, "Visible"=w779) -> (error out=w785:errorcluster)  [unwired: 1 in, 1 out]
        n215 = property on="Target Field (T)" class="DigNum (strict)"(error in=w785, "Visible"=w779) -> (error out=w784:errorcluster)  [unwired: 1 in, 1 out]
        n216 = Not(x=w779) -> (.not. x?=w778:bool)
        n217 = property on="Output Current (A)" class="DigNum (strict)"(error in=w784, "Visible"=w778) -> (error out=w783:errorcluster)  [unwired: 1 in, 1 out]
        n218 = property on="Magnet Current (A)" class="DigNum (strict)"(error in=w783, "Visible"=w778) -> (error out=w782:errorcluster)  [unwired: 1 in, 1 out]
        n219 = property on="Target Current (A)" class="DigNum (strict)"(error in=w782, "Visible"=w778) -> (error out=w781:errorcluster)  [unwired: 1 in, 1 out]
        n220 = property on="Target Rate (A/min)" class="DigNum (strict)"(error in=w781, "Visible"=w778) -> (error out=w780:errorcluster)  [unwired: 1 in, 1 out]
      }
    }
    n221 = Wait Until Next ms Multiple(millisecond multiple=u32 1000) -> ()  [unwired: 1 out]
  }
  "error out" <- w4
  n222 = property on="Current (A)" class="Knob (strict)"("Scale.Minimum"=w19, "Scale.Maximum"=w18) -> ()  [unwired: 2 in, 2 out]
  n223 = property on="Voltage (V)" class="Knob (strict)"("Scale.Minimum"=-10.0 ("y"), "Scale.Maximum"=10.0 ("y")) -> ()  [unwired: 2 in, 2 out]
